vi "UNIST Start Output.vi"(6 "Fluid Rate (CC/MIN)":T1, 8 "error in (no error)":errorcluster, 11 "VISA Refnum in":refnum<visa-resource-name>) -> (0 "error out":errorcluster, 3 "VISA Refnum out":refnum<visa-resource-name>)   [LabVIEW 2023]
uses:
  Type Definitions/UNIST Fluid Rate.ctl
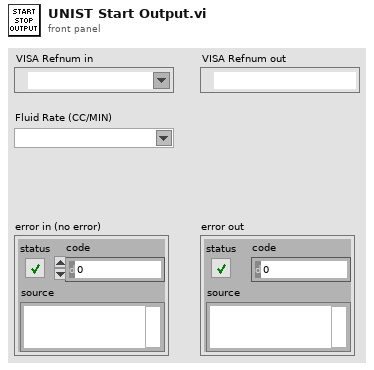
[diagram p1: front panel]
types:
  T1 = typedef "UNIST Fluid Rate.ctl" = string
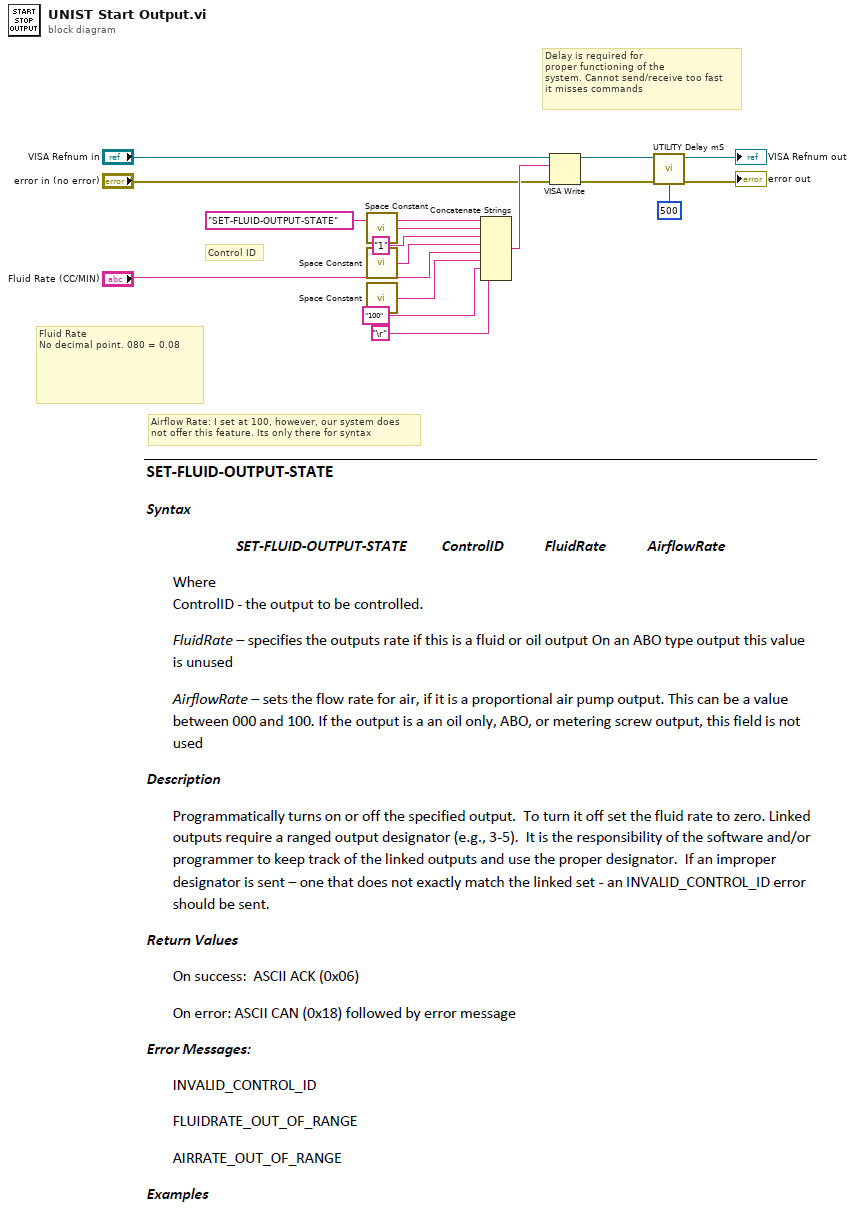
[diagram p0: block diagram]
diagram:
  # "Delay is required for \nproper functioning of the \nsystem. Cannot send/receive too fast\nit misses commands"
  # "Airflow Rate: I set at 100, however, our system does\nnot offer this feature. Its only there for syntax"
  # "Fluid Rate\nNo decimal point. 080 = 0.08"
  # "Control ID"
  n1 = call <vilib>:"Space Constant.vi"() -> ("String"=w7:string)
  n2 = call <vilib>:"Space Constant.vi"() -> ("String"=w8:string)
  n3 = call <vilib>:"Space Constant.vi"() -> ("String"=w9:string)
  n4 = Concatenate Strings("SET-FLUID-OUTPUT-STATE" ("write buffer"), w7, "1" ("string"), w8, "Fluid Rate (CC/MIN)", w9, "100" ("string"), "\r") -> (w10:string)
  n5 = VISA Write(VISA resource name="VISA Refnum in", write buffer=w10, error in (no error)="error in (no error)") -> (VISA resource name out=→"VISA Refnum out":refnum<visa-resource-name>, error out=w2:errorcluster)  [unwired: 1 out]
  n6 = call "UTILITY Delay mS.vi"("Error In"=w2, "milliseconds to wait"=u32 500) -> ("Error Out"=→"error out":errorcluster)  [unwired: 13 in]
